vi "Constructor.vi"(8 "error in (no error)":errorcluster, 11 "Observer in":refnum<class "Observer.lvclass">) -> (0 "error out":errorcluster, 2 "ObserverNotifierReference":refnum<notifier>, 3 "Observer out":refnum<class "Observer.lvclass">)   [LabVIEW 2013, in "Observer.lvclass"]
uses:
  Observer.lvclass
  Observer.lvclass/Observer.ctl
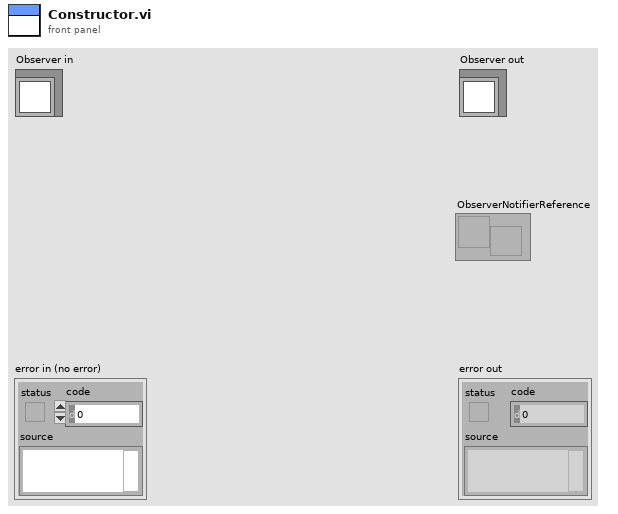
[diagram p1: front panel]
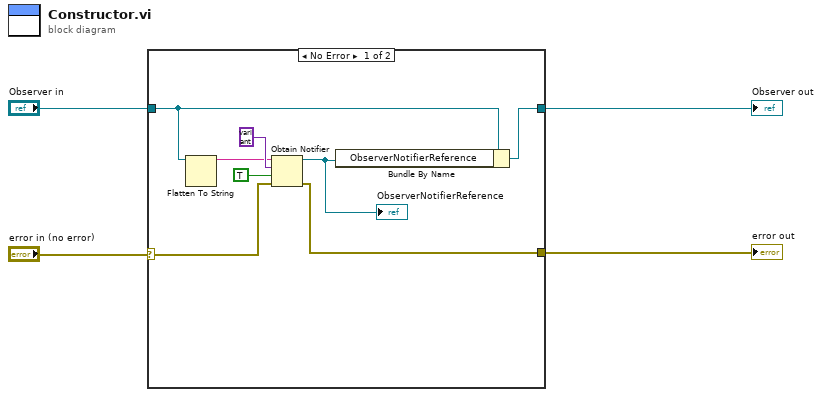
[diagram p0: block diagram]
diagram:
  n1 = case shown="No Error" "error in (no error)" {
    selector: "error in (no error)" -> [w12 w14]
    tunnel: [w8 w14] -> w2
    tunnel: [w10 w13] -> w3
    tunnel: "Observer in" -> [w6 w13]
    frame No Error {
      n2 = Flatten To String(anything=w6) -> (data string=w5:string)  [unwired: 3 in, 2 out]
      n3 = Obtain Notifier(name (unnamed)=w5, notification data type=variant ("Variant"), create if not found? (T)=TRUE, error in (no error)=w12) -> (notifier out=w11:refnum<notifier>, error out=w8:errorcluster)  [unwired: 1 out]
      "ObserverNotifierReference" <- w11
      n4 = Bundle By Name(cluster=w6, "ObserverNotifierReference"=w11) -> (w10:refnum<class "Observer.lvclass">)
    }
    frame Error {
    }
  }
  "error out" <- w2
  "Observer out" <- w3
